vi "GdsLanguage_SelectLangaugeDialog.vi"(5 "error in (no error)":errorcluster) -> (14 "SelectedLanguage":T2=enum."en", 19 "error out":errorcluster)   [LabVIEW 2020]
doc: "Sets the current and backup languages, validates these languages (checks that \nthere are non-empty strings for all StringID entries), and load the translated strings into class memory for later use in the application."
uses:
  GdsLanguage_LanguageID.ctl
  private/GdsLanguage_ChecksumCheckType.ctl
panel:
  in  "_SelectLanguage":u16(ring) caption="Välj språk" items=["English", "Swedish"]
  in  "_Cancel":bool
  in  "_OK":bool
  in  "_SelectLanguage2":T1(ring) caption="Choose language"
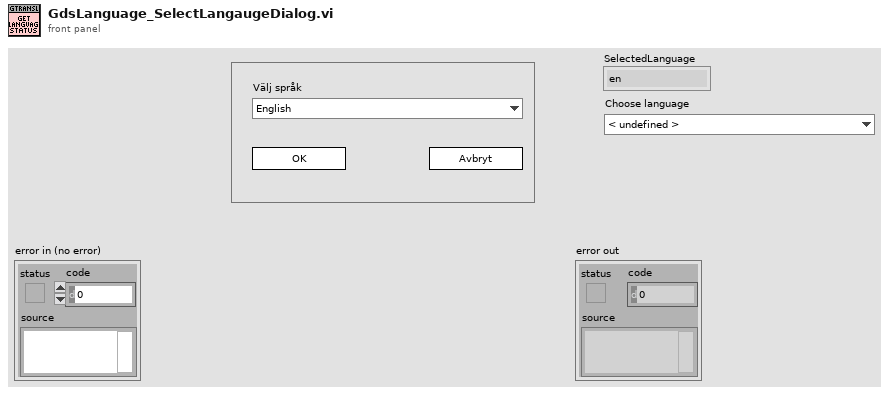
[diagram p1: front panel]
types:
  T1 = enum16{"< undefined >", "Afar", "Abkhazian", "Afrikaans", "Amharic", "Arabic", "Assamese", "Aymara", "Azerbaijani", "Bashkir", "Belarusian", "Bulgarian", "Bihari", "Bislama", "Bengali", "Tibetan", "Breton", "Catalan; Valencian", "Corsican", "Czech", "Welsh", "Danish", "German", "Dzongkha", "Greek, Modern (1453-)", "English", "Esperanto", "Spanish; Castilian", "Estonian", "Basque", "Persian", "Finnish", "Fijian", "Faroese", "French", "Western Frisian", "Irish", "Gaelic; Scottish Gaelic", "Galician", "Guarani", "Gujarati", "Manx", "Hausa", "Hebrew", "Hindi", "Croatian", "Hungarian", "Armenian", "Interlingua (International Auxiliary Language Association)", "Indonesian", "Interlingue", "Inupiaq", "Icelandic", "Italian", "Inuktitut", "Japanese", "Javanese", "Georgian", "Kazakh", "Kalaallisut; Greenlandic", "Khmer", "Kannada", "Korean", "Kashmiri", "Kurdish", "Kirghiz", "Latin", "Limburgan; Limburger; Limburgish", "Lingala", "Lao", "Lithuanian", "Latvian", "Malagasy", "Maori", "Macedonian", "Malayalam", "Mongolian", "Moldavian", "Marathi", "Malay", "Maltese", "Burmese", "Nauru", "Nepali", "Dutch; Flemish", "Norwegian", "Occitan (post 1500); Provençal", "Oromo", "Oriya", "Panjabi; Punjabi", "Polish", "Pushto", "Portuguese", "Quechua", "Raeto-Romance", "Rundi", "Romanian", "Russian", "Kinyarwanda", "Sanskrit", "Sindhi", "Sango", "", "Sinhala; Sinhalese", "Slovak", "Slovenian", "Samoan", "Shona", "Somali", "Albanian", "Serbian", "Swati", "Sotho, Southern", "Sundanese", "Swedish", "Swahili", "Tamil", "Telugu", "Tajik", "Thai", "Tigrinya", "Turkmen", "Tagalog", "Tswana", "Tonga (Tonga Islands)", "Turkish", "Tsonga", "Tatar", "Twi", "Uighur; Uyghur", "Ukrainian", "Urdu", "Uzbek", "Vietnamese", "Volapük", "Wolof", "Xhosa", "Yiddish", "Yoruba", "Chinese", "Zulu"}
  T2 = typedef "GdsLanguage_LanguageID.ctl" = enum16{"< undefined >", "aa", "ab", "af", "am", "ar", "as", "ay", "az", "ba", "be", "bg", "bh", "bi", "bn", "bo", "br", "ca", "co", "cs", "cy", "da", "de", "dz", "el", "en", "eo", "es", "et", "eu", "fa", "fi", "fj", "fo", "fr", "fy", "ga", "gd", "gl", "gn", "gu", "gv", "ha", "he", "hi", "hr", "hu", "hy", "ia", "id", "ie", "ik", "is", "it", "iu", "ja", "jv", "ka", "kk", "kl", "km", "kn", "ko", "ks", "ku", "ky", "la", "li", "ln", "lo", "lt", "lv", "mg", "mi", "mk", "ml", "mn", "mo", "mr", "ms", "mt", "my", "na", "ne", "nl", "no", "oc", "om", "or", "pa", "pl", "ps", "pt", "qu", "rm", "rn", "ro", "ru", "rw", "sa", "sd", "sg", "sh", "si", "sk", "sl", "sm", "sn", "so", "sq", "sr", "ss", "st", "su", "sv", "sw", "ta", "te", "tg", "th", "ti", "tk", "tl", "tn", "to", "tr", "ts", "tt", "tw", "ug", "uk", "ur", "uz", "vi", "vo", "wo", "xh", "yi", "yo", "zh", "zu"}
  T3 = cluster{"PreLanguage":T2, "Language":T2, "NoOfLangaugeStrings":i32, "NoOfLanuageStringsCurrentLanguageHas":i32}
  T4 = typedef "GdsLanguage_ChecksumCheckType.ctl" = enum16{"NoControl", "CheckChecksum", "AddChecksum"}
  T5 = enum32{"None", "Stop", "Question", "Exclamation", "Information"}
  T6 = typedef "GdsLanguage_ObjectAttributes.ctl" = cluster{"Language":T2, "TranslatedStrings":string[], "StringIDArray":string[], "LanguageFilesDirectory":path, "AvailableLanguages":T2[]}
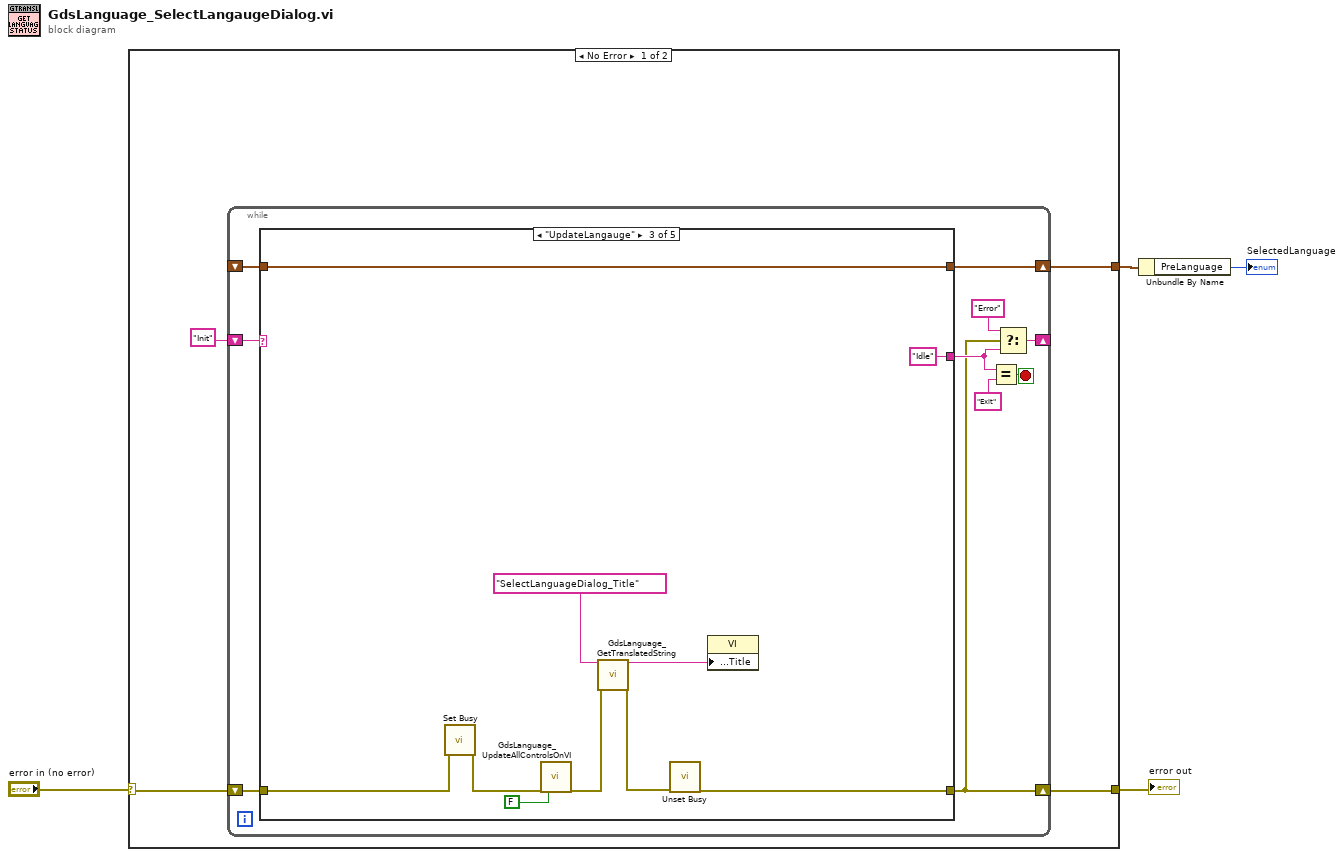
[diagram p0: block diagram]
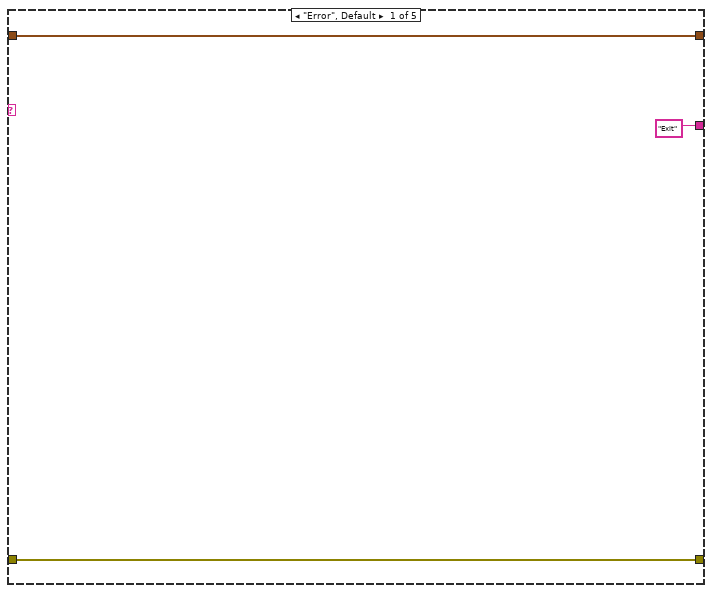
[diagram p2: hidden frame]
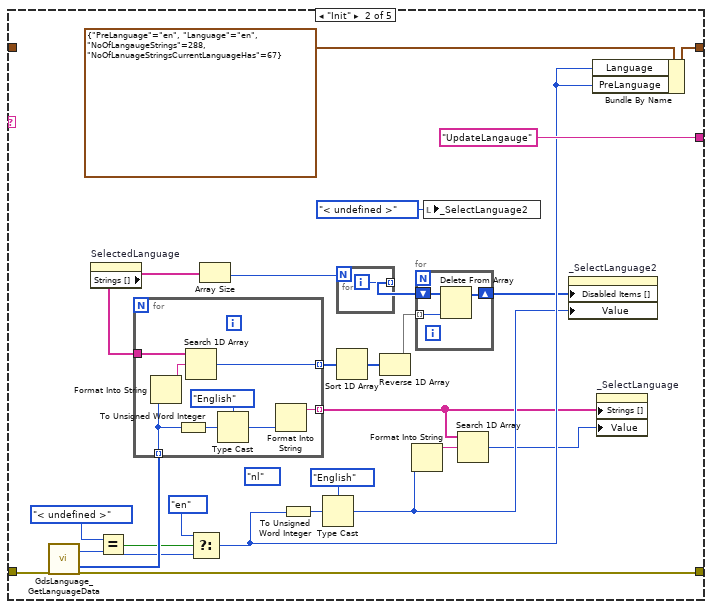
[diagram p3: hidden frame]
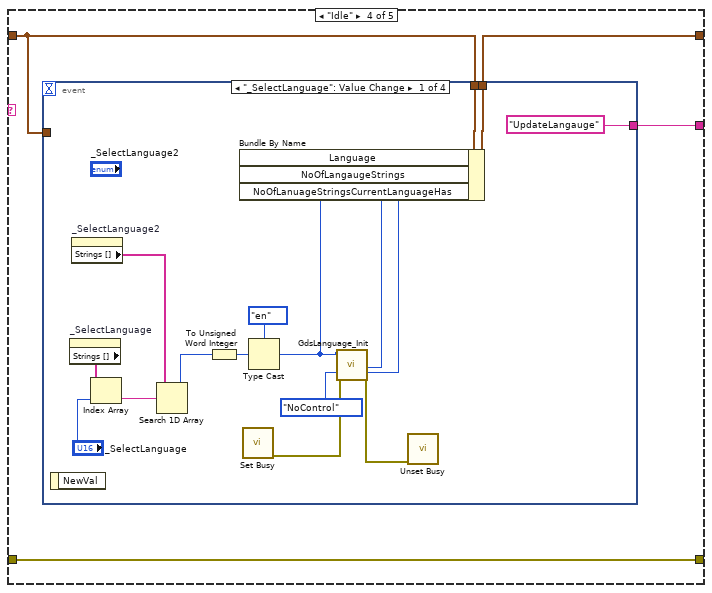
[diagram p4: hidden frame]
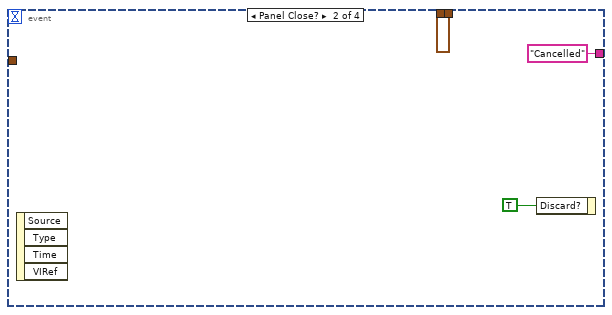
[diagram p5: hidden frame]
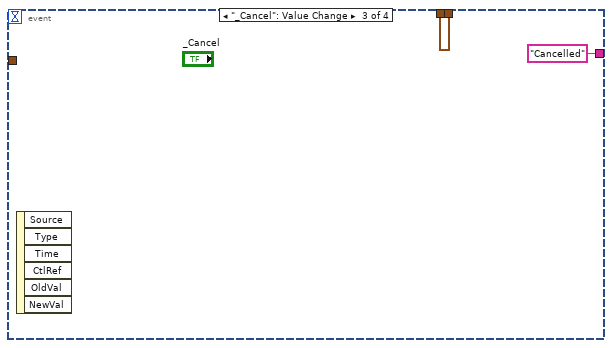
[diagram p6: hidden frame]
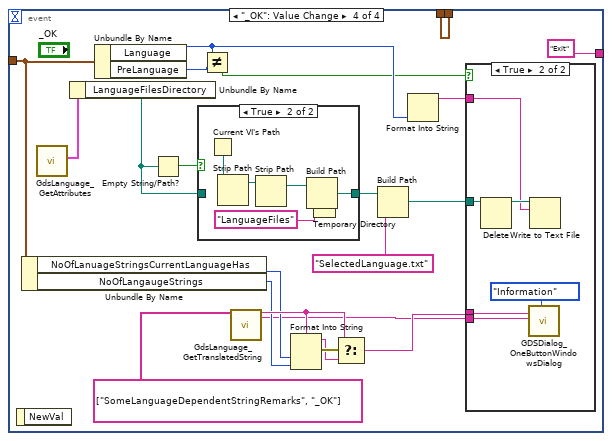
[diagram p7: hidden frame]
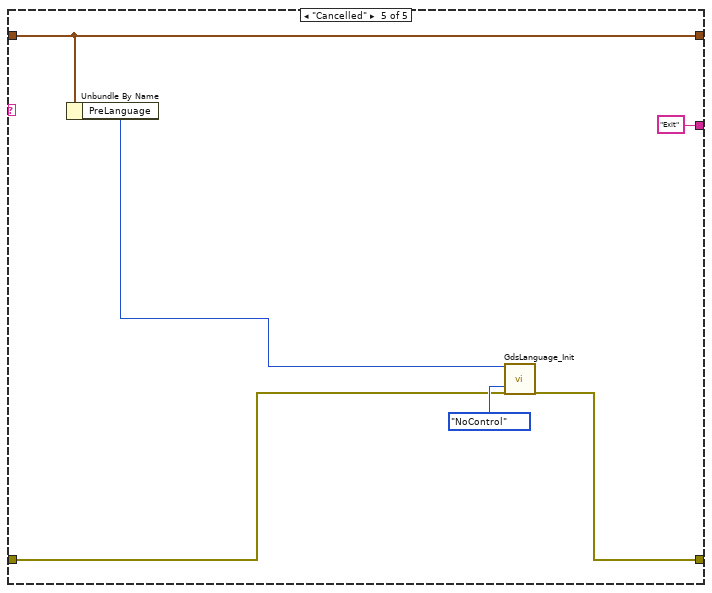
[diagram p10: hidden frame]
diagram:
  n1 = case shown="No Error" "error in (no error)" {
    selector: "error in (no error)" -> [w7 w133]
    tunnel: [w6 w133] -> w3
    tunnel: [w5 _] -> w2
    frame No Error {
      n2 = while {
        shift-right: [w9] -> w6
        shift-left: w7 -> [w18]
        shift-right: [w16] -> _
        shift-left: "Init" -> [w17]
        shift-right: [w11] -> w5
        shift-left: _ -> [w10]
        stop <- w15 stop-if-true
        n3 = case shown="\"UpdateLangauge\"" w17 {
          tunnel: w18 -> [w21 w39 w63 w72 w129]
          tunnel: ["Exit" "UpdateLangauge" "Idle" w71 "Exit"] -> w12
          tunnel: [w19 w29 w66 w70 w131] -> w11
          tunnel: w10 -> [w19 _ w66 w69 w131]
          tunnel: [w21 w38 w60 w72 w128] -> w9
          frame "Error", Default {
          }
          frame "Init" {
            (unwired) GdsLanguage_LanguageID."nl" ("SelectedLanguage")
            n4 = call "GdsLanguage_GetLanguageData.vi"("error in (no error)"=w39) -> ("Language"=w31:T2, "FoundLanguages"=w35:T2[], "error out"=w38:errorcluster)  [unwired: 14 in, 2 out]
            n5 = property on="SelectedLanguage" class="Enum (strict)"() -> ("Strings []"=w40:string[])  [unwired: 2 in, 2 out]
            n6 = Equal?(x=GdsLanguage_LanguageID."< undefined >" ("SelectedLanguage"), y=w31) -> (x = y?=w33:bool)
            n7 = for {
              tunnel: w40 -> [w58]
              tunnel: [w56] -> w44 mode=indexing
              tunnel: w35 -> [w53] mode=indexing
              tunnel: [w51] -> w24 mode=indexing
              n8 = Format Into String(w53) -> (resulting string=w57:string)  [unwired: 3 in, 1 out]
              n9 = To Unsigned Word Integer(number=w53) -> (unsigned 16bit integer=w55:u16)
              n10 = Search 1D Array(1D array=w58, element=w57) -> (index of element=w56:i32)  [unwired: 1 in]
              n11 = Type Cast(type=T1."English", x=w55) -> (*(type *) &x=w52:T1)
              n12 = Format Into String(w52) -> (resulting string=w51:string)  [unwired: 3 in, 1 out]
            }
            n13 = Select(t=GdsLanguage_LanguageID."en" ("SelectedLanguage"), s=w33, f=w31) -> (s? t:f=w28:T2)
            n14 = Array Size(array=w40) -> (size(s)=w45:i32)
            n15 = To Unsigned Word Integer(number=w28) -> (unsigned 16bit integer=w36:u16)
            n16 = Type Cast(type=T1."English", x=w36) -> (*(type *) &x=w25:T1)
            n17 = for {
              N: w45 -> [_]
              tunnel: [w50] -> w42 mode=indexing
              i -> [w50]
            }
            n18 = Sort 1D Array(array=w44) -> (sorted array=w43:i32[])
            n19 = Reverse 1D Array(array=w43) -> (reversed array=w41:i32[])
            n20 = Format Into String(w25) -> (resulting string=w23:string)  [unwired: 3 in, 1 out]
            n21 = for {
              shift-right: [w48] -> w27
              shift-left: w42 -> [w49]
              tunnel: w41 -> [w47] mode=indexing
              n22 = Delete From Array(array=w49, index=w47) -> (array with subset deleted=w48:i32[])  [unwired: 1 in, 1 out]
            }
            n23 = local write "_SelectLanguage2"(T1."< undefined >" ("_SelectLanguage")) -> ()
            n24 = Search 1D Array(1D array=w24, element=w23) -> (index of element=w22:i32)  [unwired: 1 in]
            n25 = property on="_SelectLanguage2" class="Enum (strict)"("Disabled Items []"=w27, "Value"=w25) -> ()  [unwired: 2 in, 2 out]
            n26 = Bundle By Name(cluster=T3 {"PreLanguage"=enum."en", "Language"=enum."en", "NoOfLangaugeStrings"=288, "NoOfLanuageStringsCurrentLanguageHas"=67}, "Language"=w28, "PreLanguage"=w28) -> (w29:T3)
            n27 = property on="_SelectLanguage" class="Ring (strict)"("Strings []"=w24, "Value"=w22) -> ()  [unwired: 2 in, 2 out]
          }
          frame "UpdateLangauge" {
            n28 = call <vilib>:"Set Busy.vi"("error in (no error)"=w63) -> ("error out"=w62:errorcluster)  [unwired: 9 in, 1 out]
            n29 = call "GdsLanguage_UpdateAllControlsOnVI.vi"("error in (no error)"=w62, "CreateLanguageFile(Use this to create a languageFile)"=FALSE) -> ("error out"=w61:errorcluster)  [unwired: 16 in, 1 out]
            n30 = call "GdsLanguage_GetTranslatedString.vi"("StringID(s)"="SelectLanguageDialog_Title", "error in (no error)"=w61) -> ("FirstStringOut"=w64:string, "error out"=w59:errorcluster)  [unwired: 14 in, 2 out]
            n31 = call <vilib>:"Unset Busy.vi"("error in (no error)"=w59) -> ("error out"=w60:errorcluster)  [unwired: 10 in]
            n32 = property class="VI"("Front Panel.Title"=w64) -> ()  [unwired: 2 in, 2 out]
          }
          frame "Idle" {
            n33 = event shown="[0] \"_SelectLanguage\": Value Change" {
              selector: _ -> [_ _ _ _]
              dyn-events: _ -> [_ _ _ _]
              timeout: _ -> [_ _ _ _]
              tunnel: ["UpdateLangauge" "Cancelled" "Cancelled" "Exit"] -> w71
              tunnel: w69 -> [w85 w89 w92 w106]
              tunnel: [w84 w89 w92 w106] -> w70
              tunnel: w69 -> [_ _ _ w102]
              event "_SelectLanguage": Value Change {
                n34 = event-data() -> ()  [unwired: 1 in, 1 out]
                n35 = property on="_SelectLanguage" class="Ring (strict)"() -> ("Strings []"=w79:string[])  [unwired: 2 in, 2 out]
                n36 = property on="_SelectLanguage2" class="Enum (strict)"() -> ("Strings []"=w77:string[])  [unwired: 2 in, 2 out]
                n37 = Index Array(array=w79, index="_SelectLanguage") -> (element=w76:string)
                n38 = Search 1D Array(1D array=w77, element=w76) -> (index of element=w75:i32)  [unwired: 1 in]
                n39 = To Unsigned Word Integer(number=w75) -> (unsigned 16bit integer=w88:u16)
                n40 = call <vilib>:"Set Busy.vi"() -> ("error out"=w74:errorcluster)  [unwired: 10 in, 1 out]
                n41 = Type Cast(type=GdsLanguage_LanguageID."en" ("SelectedLanguage"), x=w88) -> (*(type *) &x=w82:T2)
                n42 = call "GdsLanguage_Init.vi"("PrimaryLanguage"=w82, "ChesumControl"=GdsLanguage_ChecksumCheckType."NoControl", "error in (no error)"=w74) -> ("NoOfLangaugeStrings"=w81:i32, "NoOfLanuageStringsCurrentLanguageHas"=w80:i32, "error out"=w73:errorcluster)  [unwired: 13 in, 1 out]
                n43 = Bundle By Name(cluster=w85, "Language"=w82, "NoOfLangaugeStrings"=w81, "NoOfLanuageStringsCurrentLanguageHas"=w80) -> (w84:T3)
                n44 = call <vilib>:"Unset Busy.vi"("error in (no error)"=w73) -> ()  [unwired: 10 in, 1 out]
              }
              event Panel Close? {
                n45 = event-data() -> ()  [unwired: 1 in, 4 out]
                n46 = event-data("Discard?"=TRUE) -> ()  [unwired: 1 in, 1 out]
              }
              event "_Cancel": Value Change {
                n47 = event-data() -> ()  [unwired: 1 in, 6 out]
              }
              event "_OK": Value Change {
                n48 = event-data() -> ()  [unwired: 1 in, 1 out]
                n49 = Unbundle By Name(w102) -> ("NoOfLanuageStringsCurrentLanguageHas"=w101:i32, "NoOfLangaugeStrings"=w100:i32)
                n50 = call "GdsLanguage_GetAttributes.vi"() -> ("Attributes"=w110:T6)  [unwired: 18 in, 1 out]
                n51 = Unbundle By Name(w110) -> ("LanguageFilesDirectory"=w95:path)
                n52 = Unbundle By Name(w102) -> ("Language"=w97:T2, "PreLanguage"=w96:T2)
                n53 = Empty String/Path?(string/path=w95) -> (empty?=w112:bool)
                n54 = case shown="True" w112 {
                  tunnel: [w121 w123] -> _
                  tunnel: w95 -> [w121 _]
                  frame False {
                  }
                  frame True {
                    n55 = Current VI's Path() -> (path=w122:path)
                    n56 = Strip Path(path=w122) -> (stripped path=w126:path)  [unwired: 1 out]
                    n57 = Strip Path(path=w126) -> (stripped path=w125:path)  [unwired: 1 out]
                    n58 = Build Path(base path=w125, name or relative path="LanguageFiles") -> (appended path=w123:path)
                  }
                }
                n59 = Not Equal?(x=w97, y=w96) -> (x != y?=w94:bool)
                n60 = call "GdsLanguage_GetTranslatedString.vi"("StringID(s)"=string[] ["SomeLanguageDependentStringRemarks", "_OK"]) -> ("FirstStringOut"=w104:string, "SecondStringOut"=w98:string)  [unwired: 15 in, 2 out]
                n61 = Format Into String(format string=w104, w101, w100) -> (resulting string=w103:string, error out=w105:errorcluster)  [unwired: 2 in]
                n62 = Temporary Directory() -> (w113:path)
                n63 = Select(t=w104, s=w105, f=w103) -> (s? t:f=w99:string)
                n64 = Build Path(base path=w113, name or relative path="SelectedLanguage.txt") -> (appended path=w109:path)
                n65 = Format Into String(w97) -> (resulting string=w108:string)  [unwired: 3 in, 1 out]
                n66 = case shown="True" w94 {
                  tunnel: w109 -> [_ w120]
                  tunnel: w108 -> [_ w118]
                  tunnel: w99 -> [_ w116]
                  tunnel: w98 -> [_ w115]
                  frame False {
                  }
                  frame True {
                    n67 = Delete(path (use dialog)=w120) -> (deleted path=w119:path)  [unwired: 4 in, 2 out]
                    n68 = call "GDSDialog_OneButtonWindowsDialog.vi"("UserText"=w116, "ButtonName"=w115, "Icon"=T5."Information") -> ()  [unwired: 14 in, 3 out]
                    n69 = Write to Text File(file (use dialog)=w119, text=w118) -> ()  [unwired: 2 in, 3 out]
                  }
                }
              }
            }
          }
          frame "Cancelled" {
            n70 = Unbundle By Name(w131) -> ("PreLanguage"=w127:T2)
            n71 = call "GdsLanguage_Init.vi"("PrimaryLanguage"=w127, "ChesumControl"=GdsLanguage_ChecksumCheckType."NoControl", "error in (no error)"=w129) -> ("error out"=w128:errorcluster)  [unwired: 13 in, 3 out]
          }
        }
        n72 = Equal?(x=w12, y="Exit") -> (x = y?=w15:bool)
        n73 = Select(t="Error", s=w9, f=w12) -> (s? t:f=w16:string)
      }
    }
    frame Error {
    }
  }
  "error out" <- w3
  n74 = Unbundle By Name(w2) -> ("PreLanguage"=→"SelectedLanguage":T2)
